vi "Get Status Channels.vi"(8 "error in":errorcluster, 11 "section reference in":T1 format="%.0x") -> (0 "error out":errorcluster, 2 "status channels":T1[](array[typedef]) format="%.0x", 3 "section reference out":T1 format="%.0x", 4 "found?":bool)   [LabVIEW 2020, in "Ballard MIL-STD-1553 Scripting.lvlib"]
uses:
  Ballard MIL-STD-1553 Scripting.lvlib
  <vilib>/NI VeriStand/Custom Device API/Custom Device Item Ref.ctl
  Constants.vi
  <vilib>/NI VeriStand/Custom Device Tools/Custom Device Utility Library/NI VeriStand - Search for All Items by GUID.vi
  <vilib>/NI VeriStand/Custom Device Tools/Custom Device Utility Library/Custom Device Utility Library.lvlib
  <vilib>/NI VeriStand/Custom Device API/Custom Device API.lvlib
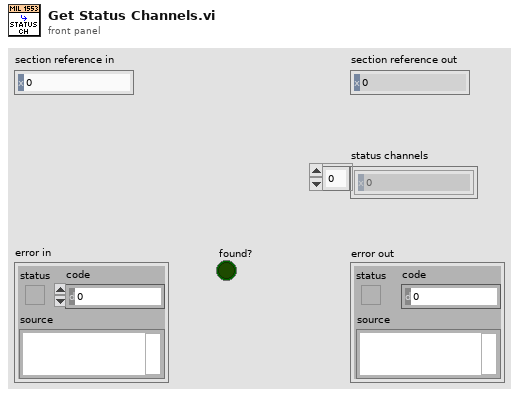
[diagram p1: front panel]
types:
  T1 = typedef "Custom Device API.lvlib/Custom Device Item Ref.ctl" = u64
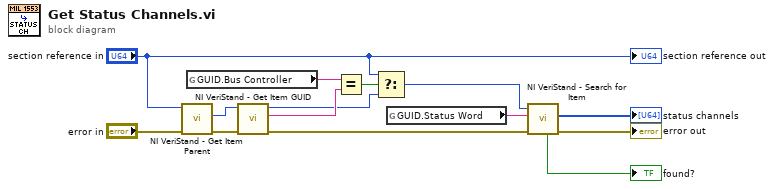
[diagram p0: block diagram]
diagram:
  n1 = call <vilib>:"NI VeriStand - Get Item Parent.vi"("error in (no error)"="error in", "Item Ref in"="section reference in") -> ("error out"=w6:errorcluster, "Parent Ref"=w7:T1)  [unwired: 6 in, 2 out]
  n2 = global read "Constants.vi" "GUID.Bus Controller"() -> (w9:string)
  n3 = call <vilib>:"NI VeriStand - Get Item GUID.vi"("error in (no error)"=w6, "Item Ref in"=w7) -> ("error out"=w1:errorcluster, "GUID"=w10:string, "Item Ref out"=w3:T1)  [unwired: 7 in]
  n4 = Equal?(x=w9, y=w10) -> (x = y?=w5:bool)
  n5 = Select(t="section reference in", s=w5, f=w3) -> (s? t:f=w2:T1)
  n6 = global read "Constants.vi" "GUID.Status Word"() -> (w13:string)
  n7 = call-poly <vilib>:"NI VeriStand - Search for Item.vi"("error in"=w1, "Item GUID"=w13, "Section Ref in"=w2) -> ("error out"=→"error out":errorcluster, "Item Refs"=→"status channels":T1[], "Found"=→"found?":bool)  [unwired: 5 in, 1 out]
  "section reference out" <- "section reference in"
